vi "Begin.vi"(11 "Image Size":T1=enum."160x120") -> (0 "error out":errorcluster)   [LabVIEW 2012]
doc: "Called before other user functions, this VI is expected to open initial I/O refnums, load in file data, and do all program initialization. Notice that the <B>error out</B> terminal is simply used for data flow. Wiring it to other structures or subVIs ensures that this VI runs first."
uses:
  <vilib>/Rock Robotics/WPI/Camera/WPI_CameraImageSize.ctl
  <vilib>/Rock Robotics/WPI/Camera/WPI_CameraWhite Balance Values.ctl
  <vilib>/Rock Robotics/WPI/Camera/WPI_CameraExposure Values.ctl
  <vilib>/Rock Robotics/WPI/Camera/WPI_CameraFrameRate.ctl
  <vilib>/Rock Robotics/WPI/DriverStation/WPI_DriverStationRobotMode2.ctl
  <vilib>/Rock Robotics/WPI/Joystick/WPI_JoystickDeviceEnum.ctl
  <vilib>/Rock Robotics/WPI/CAN/Jaguar/SubVIs/WPI_CANJaguar_ControlMode.ctl
  <vilib>/Rock Robotics/WPI/CAN/Jaguar/SubVIs/WPI_CANJaguar_SpeedReference.ctl
  <vilib>/Rock Robotics/WPI/CAN/Jaguar/SubVIs/WPI_CANJaguar_PositionReference.ctl
  Robot Global Data.vi
  <vilib>/Rock Robotics/WPI/MotorControl/WPI_MotorControlOpenCANJaguar.vi
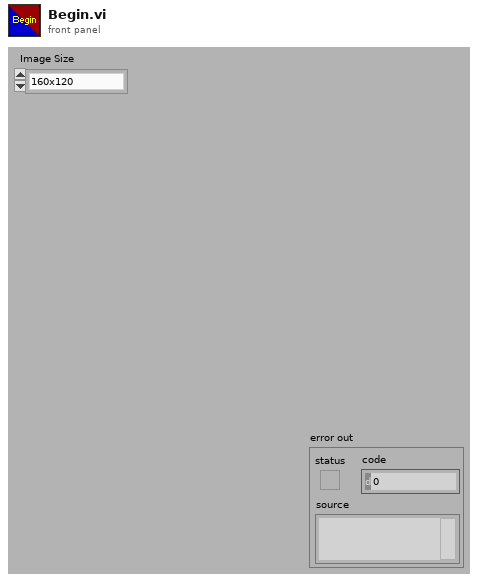
[diagram p1: front panel]
types:
  T1 = typedef "WPI_CameraImageSize.ctl" = enum16{"640x480", "320x240", "160x120"}
  T2 = typedef "WPI_JoystickDeviceEnum.ctl" = enum16{"USB 1", "USB 2", "USB 3", "USB 4", "Kinect 1", "Kinect 2"}
  T3 = typedef "WPI_CANJaguar_PositionReference.ctl" = u8
  T4 = typedef "WPI_CANJaguar_ControlMode.ctl" = enum8{"Percent VBus", "Current", "Speed", "Position", "Voltage"}
  T5 = typedef "WPI_CANJaguar_SpeedReference.ctl" = u8
  T6 = typedef "WPI_DriverStationRobotMode2.ctl" = enum16{"Autonomous Disabled", "Autonomous Enabled", "Teleop Disabled", "Teleop Enabled", "Timeout", "Finish", "Test Disabled", "Test Enabled"}
  T7 = typedef "WPI_CameraFrameRate.ctl" = u32
  T8 = typedef "WPI_CameraExposure Values.ctl" = enum16{"Auto", "Flicker-free 50 Hz", "Flicker-free 60 Hz", "Hold current"}
  T9 = typedef "WPI_CameraWhite Balance Values.ctl" = enum16{"Auto", "Fixed indoor", "Fixed outdoor 1", "Fixed outdoor 2", "Fixed fluorescent 1", "Fixed fluorescent 2", "Hold current"}
  T10 = typedef "WPI_MotorControlDeviceRef.ctl" = cluster{"DeviceStatus":errorcluster, "Type":enum16{"PWM", "CAN"}, "PWM":cluster{"Digital Module":T11, "PWM Channel":T12, "DeadBand":T13}, "CAN":cluster{"Device Number":u8, "Control Mode":T4, "Semaphore":T14, "Max Vout":dbl}, "Invert":bool, "TransformRef":T15, "InvTransformRef":T15}
  T11 = typedef "FPGA_TypedefDigitalModule.ctl" = enum16{"Digital Module 1", "Digital Module 2"}
  T12 = typedef "FPGA_DIOPWMChannel.ctl" = enum8{"PWM 1", "PWM 2", "PWM 3", "PWM 4", "PWM 5", "PWM 6", "PWM 7", "PWM 8", "PWM 9", "PWM 10", "Invalid"}
  T13 = typedef "WPI_PWMDeadband.ctl" = cluster{"Name":string, "maxPositivePwm":i32, "minPositivePwm":i32, "centerPwm":i32, "maxNegativePwm":i32, "minNegativePwm":i32, "angularRange":u16}
  T14 = typedef "Semaphore RefNum" = refnum<k1>
  T15 = typedef "WPI_PWMTransform_ConPane.ctl" = refnum<vi>
  T16 = typedef "WPI_JoystickDevRef.ctl" = cluster{"Device":T2}
  T17 = typedef "WPI_CameraDevRef.ctl" = cluster{"Camera Address":string, "CameraStatus":errorcluster, "Acquire Image Notifier":refnum<notifier>}
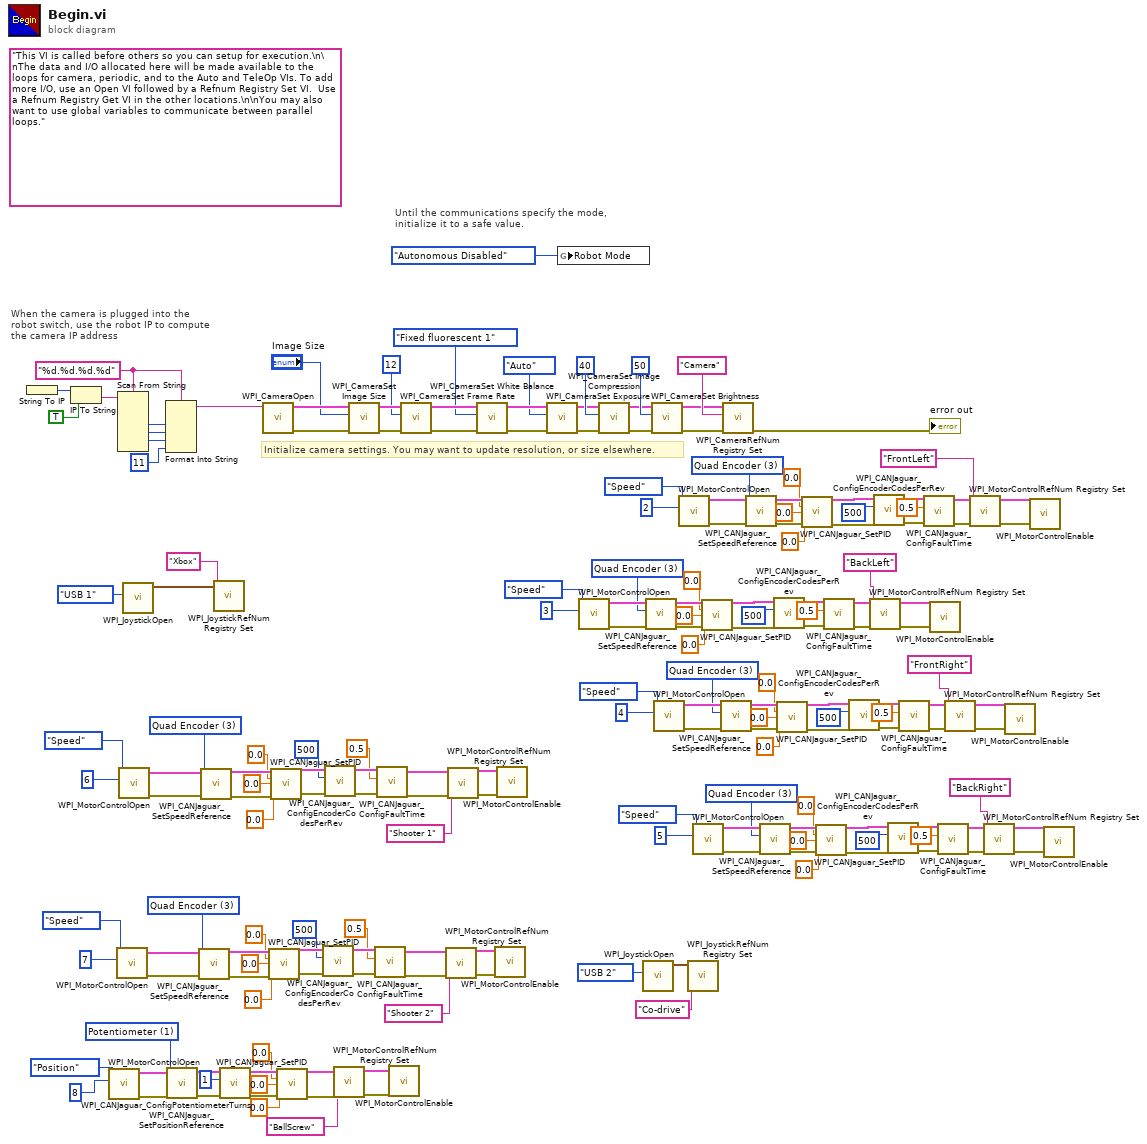
[diagram p0: block diagram]
diagram:
  w17 = T3 1 items=["Quad Encoder"=0, "Potentiometer"=1, "None"=255] ("Position Reference")
  w38 = T5 3 items=["Encoder"=0, "Inv Encoder"=2, "Quad Encoder"=3, "None"=255] ("Speed Reference")
  w59 = T5 3 items=["Encoder"=0, "Inv Encoder"=2, "Quad Encoder"=3, "None"=255] ("Speed Reference")
  w65 = T5 3 items=["Encoder"=0, "Inv Encoder"=2, "Quad Encoder"=3, "None"=255] ("Speed Reference")
  w86 = T5 3 items=["Encoder"=0, "Inv Encoder"=2, "Quad Encoder"=3, "None"=255] ("Speed Reference")
  w107 = T5 3 items=["Encoder"=0, "Inv Encoder"=2, "Quad Encoder"=3, "None"=255] ("Speed Reference")
  w143 = T5 3 items=["Encoder"=0, "Inv Encoder"=2, "Quad Encoder"=3, "None"=255] ("Speed Reference")
  w154 = "%d.%d.%d.%d" ("format string")
  (unwired) "This VI is called before others so you can setup for execution.\n\nThe data and I/O allocated here will be made available to the loops for camera, periodic, and to the Auto and TeleOp VIs. To add more I/O, use an Open VI followed by a Refnum Registry Set VI.  Use a Refnum Registry Get VI in the other locations.\n\nYou may also want to use global variables to communicate between parallel loops."
  # "Until the communications specify the mode,\ninitialize it to a safe value."
  # "When the camera is plugged into the\nrobot switch, use the robot IP to compute\nthe camera IP address"
  # "Initialize camera settings. You may want to update resolution, or size elsewhere."
  n1 = String To IP() -> (0:w161:u32)  [unwired: 1 in]
  n2 = IP To String(1:TRUE ("dot notation? (F)"), 2:w161) -> (0:w159:string)
  n3 = call-poly <vilib>:"WPI_MotorControlOpen.vi"("Device Number"=u8 8, "Control Mode"=WPI_CANJaguar_ControlMode."Position") -> ("error out"=w19:errorcluster, "MotorControlDeviceRef"=w18:T10)  [unwired: 8 in]
  n4 = call-poly <vilib>:"WPI_MotorControlOpen.vi"("Device Number"=u8 7, "Control Mode"=WPI_CANJaguar_ControlMode."Speed") -> ("error out"=w39:errorcluster, "MotorControlDeviceRef"=w40:T10)  [unwired: 8 in]
  n5 = Scan From String(format string=w154, input string=w159) -> (output 1=w158:i32, output 2=w157:i32, output 3=w156:i32)  [unwired: 7 in, 3 out]
  n6 = call-poly <vilib>:"WPI_MotorControlOpen.vi"("Device Number"=u8 6, "Control Mode"=WPI_CANJaguar_ControlMode."Speed") -> ("error out"=w60:errorcluster, "MotorControlDeviceRef"=w61:T10)  [unwired: 8 in]
  n7 = call <vilib>:"WPI_JoystickOpen.vi"("JoystickDevice"=WPI_JoystickDeviceEnum."USB 1") -> ("JoystickDevRef"=w150:T16)  [unwired: 10 in]
  n8 = Format Into String(format string=w154, w158, w157, w156, 11 ("Compression")) -> (resulting string=w152:string)  [unwired: 2 in, 1 out]
  n9 = call <vilib>:"WPI_CANJaguar_SetPositionReference.vi"("error in (no error)"=w19, "Position Reference"=w17, "CAN Jaguar Ref"=w18) -> ("error out"=w16:errorcluster, "CAN Jaguar Ref Out"=w15:T10)  [unwired: 7 in]
  n10 = call <vilib>:"WPI_CANJaguar_SetSpeedReference.vi"("error in (no error)"=w39, "Speed Reference"=w38, "CAN Jaguar Ref"=w40) -> ("error out"=w36:errorcluster, "CAN Jaguar Ref Out"=w37:T10)  [unwired: 7 in]
  n11 = call <vilib>:"WPI_CANJaguar_SetSpeedReference.vi"("error in (no error)"=w60, "Speed Reference"=w59, "CAN Jaguar Ref"=w61) -> ("error out"=w57:errorcluster, "CAN Jaguar Ref Out"=w58:T10)  [unwired: 7 in]
  n12 = call <vilib>:"WPI_JoystickRefNum Registry Set.vi"("refnum name"="Xbox", "JoystickDevRef"=w150) -> ()  [unwired: 8 in, 2 out]
  n13 = call <vilib>:"WPI_CANJaguar_ConfigPotentiometerTurns.vi"("error in (no error)"=w16, "Potentiometer Turns"=u16 1, "CAN Jaguar Ref"=w15) -> ("error out"=w12:errorcluster, "CAN Jaguar Ref Out"=w13:T10)  [unwired: 7 in]
  n14 = call <vilib>:"WPI_CameraOpen.vi"("Camera Address"=w152) -> ("error out"=w173:errorcluster, "CameraDevRef"=w174:T17)  [unwired: 1 in, 8 out]
  n15 = call <vilib>:"WPI_CANJaguar_SetPID.vi"("CAN Jaguar Ref"=w37, "P"=0.0, "I"=0.0, "D"=0.0, "error in (no error)"=w36) -> ("CAN Jaguar Ref Out"=w32:T10, "error out"=w31:errorcluster)  [unwired: 9 in]
  n16 = call <vilib>:"WPI_CANJaguar_SetPID.vi"("CAN Jaguar Ref"=w58, "P"=0.0, "I"=0.0, "D"=0.0, "error in (no error)"=w57) -> ("CAN Jaguar Ref Out"=w53:T10, "error out"=w52:errorcluster)  [unwired: 9 in]
  n17 = call <vilib>:"WPI_CANJaguar_SetPID.vi"("CAN Jaguar Ref"=w13, "P"=0.0, "I"=0.0, "D"=0.0, "error in (no error)"=w12) -> ("CAN Jaguar Ref Out"=w7:T10, "error out"=w8:errorcluster)  [unwired: 9 in]
  n18 = call <vilib>:"WPI_CANJaguar_ConfigEncoderCodesPerRev.vi"("error in (no error)"=w31, "Encoder Codes Per Rev"=u16 500, "CAN Jaguar Ref"=w32) -> ("error out"=w29:errorcluster, "CAN Jaguar Ref Out"=w28:T10)  [unwired: 7 in]
  n19 = call <vilib>:"WPI_CANJaguar_ConfigEncoderCodesPerRev.vi"("error in (no error)"=w52, "Encoder Codes Per Rev"=u16 500, "CAN Jaguar Ref"=w53) -> ("error out"=w50:errorcluster, "CAN Jaguar Ref Out"=w49:T10)  [unwired: 7 in]
  n20 = call <vilib>:"WPI_MotorControlRefNum Registry Set.vi"("error in (no error)"=w8, "refnum name"="BallScrew", "MotorControlDevRef"=w7) -> ("error out"=w6:errorcluster, "MotorControlDevRef"=w5:T10)  [unwired: 7 in]
  n21 = call <vilib>:"WPI_CameraSet Image Size.vi"("error in (no error)"=w173, "Image Size"="Image Size", "CameraDevRef"=w174) -> ("error out"=w172:errorcluster, "CameraDevRef Out"=w175:T17)  [unwired: 7 out]
  n22 = call <vilib>:"WPI_CANJaguar_ConfigFaultTime.vi"("error in (no error)"=w29, "Fault Time (s)"=0.5, "CAN Jaguar Ref"=w28) -> ("error out"=w24:errorcluster, "CAN Jaguar Ref Out"=w25:T10)  [unwired: 7 in]
  n23 = call <vilib>:"WPI_CANJaguar_ConfigFaultTime.vi"("error in (no error)"=w50, "Fault Time (s)"=0.5, "CAN Jaguar Ref"=w49) -> ("error out"=w45:errorcluster, "CAN Jaguar Ref Out"=w46:T10)  [unwired: 7 in]
  n24 = call <vilib>:"WPI_MotorControlEnable.vi"("error in (no error)"=w6, "CAN Jaguar Ref"=w5) -> ()  [unwired: 8 in, 2 out]
  n25 = call <vilib>:"WPI_CameraSet Frame Rate.vi"("error in (no error)"=w172, "Frame Rate (fps)"=T7 12, "CameraDevRef"=w175) -> ("error out"=w171:errorcluster, "CameraDevRef Out"=w177:T17)  [unwired: 7 out]
  n26 = call <vilib>:"WPI_MotorControlRefNum Registry Set.vi"("error in (no error)"=w24, "refnum name"="Shooter 2", "MotorControlDevRef"=w25) -> ("error out"=w22:errorcluster, "MotorControlDevRef"=w23:T10)  [unwired: 7 in]
  n27 = call <vilib>:"WPI_MotorControlRefNum Registry Set.vi"("error in (no error)"=w45, "refnum name"="Shooter 1", "MotorControlDevRef"=w46) -> ("error out"=w43:errorcluster, "MotorControlDevRef"=w44:T10)  [unwired: 7 in]
  n28 = call <vilib>:"WPI_CameraSet White Balance.vi"("error in (no error)"=w171, "White Balance"=WPI_CameraWhite_Balance_Values."Fixed fluorescent 1", "CameraDevRef"=w177) -> ("error out"=w170:errorcluster, "CameraDevRef Out"=w176:T17)  [unwired: 7 out]
  n29 = call <vilib>:"WPI_MotorControlEnable.vi"("error in (no error)"=w22, "CAN Jaguar Ref"=w23) -> ()  [unwired: 8 in, 2 out]
  n30 = call <vilib>:"WPI_MotorControlEnable.vi"("error in (no error)"=w43, "CAN Jaguar Ref"=w44) -> ()  [unwired: 8 in, 2 out]
  n31 = call <vilib>:"WPI_CameraSet Exposure.vi"("error in (no error)"=w170, "Exposure"=WPI_CameraExposure_Values."Auto", "CameraDevRef"=w176) -> ("error out"=w169:errorcluster, "CameraDevRef Out"=w179:T17)  [unwired: 7 out]
  n32 = global write "Robot Global Data.vi" "Robot Mode"(WPI_DriverStationRobotMode2."Autonomous Disabled" ("Robot Mode")) -> ()
  n33 = call-poly <vilib>:"WPI_MotorControlOpen.vi"("Device Number"=u8 3, "Control Mode"=WPI_CANJaguar_ControlMode."Speed") -> ("error out"=w123:errorcluster, "MotorControlDeviceRef"=w124:T10)  [unwired: 8 in]
  n34 = call <vilib>:"WPI_CameraSet Image Compression.vi"("error in (no error)"=w169, "Compression"=40, "CameraDevRef"=w179) -> ("error out"=w168:errorcluster, "CameraDevRef Out"=w178:T17)  [unwired: 7 out]
  n35 = call <vilib>:"WPI_JoystickOpen.vi"("JoystickDevice"=WPI_JoystickDeviceEnum."USB 2") -> ("JoystickDevRef"=w2:T16)  [unwired: 10 in]
  n36 = call <vilib>:"WPI_CANJaguar_SetSpeedReference.vi"("error in (no error)"=w123, "Speed Reference"=w107, "CAN Jaguar Ref"=w124) -> ("error out"=w121:errorcluster, "CAN Jaguar Ref Out"=w122:T10)  [unwired: 7 in]
  n37 = call <vilib>:"WPI_CameraSet Brightness.vi"("error in (no error)"=w168, "Brightness"=50, "CameraDevRef"=w178) -> ("error out"=w166:errorcluster, "CameraDevRef Out"=w167:T17)  [unwired: 7 out]
  n38 = call-poly <vilib>:"WPI_MotorControlOpen.vi"("Device Number"=u8 4, "Control Mode"=WPI_CANJaguar_ControlMode."Speed") -> ("error out"=w102:errorcluster, "MotorControlDeviceRef"=w103:T10)  [unwired: 8 in]
  n39 = call-poly <vilib>:"WPI_MotorControlOpen.vi"("Device Number"=u8 2, "Control Mode"=WPI_CANJaguar_ControlMode."Speed") -> ("error out"=w144:errorcluster, "MotorControlDeviceRef"=w145:T10)  [unwired: 8 in]
  n40 = call <vilib>:"WPI_JoystickRefNum Registry Set.vi"("refnum name"="Co-drive", "JoystickDevRef"=w2) -> ()  [unwired: 8 in, 2 out]
  n41 = call-poly <vilib>:"WPI_MotorControlOpen.vi"("Device Number"=u8 5, "Control Mode"=WPI_CANJaguar_ControlMode."Speed") -> ("error out"=w81:errorcluster, "MotorControlDeviceRef"=w82:T10)  [unwired: 8 in]
  n42 = call <vilib>:"WPI_CANJaguar_SetPID.vi"("CAN Jaguar Ref"=w122, "P"=0.0, "I"=0.0, "D"=0.0, "error in (no error)"=w121) -> ("CAN Jaguar Ref Out"=w116:T10, "error out"=w117:errorcluster)  [unwired: 9 in]
  n43 = call <vilib>:"WPI_CANJaguar_SetSpeedReference.vi"("error in (no error)"=w102, "Speed Reference"=w86, "CAN Jaguar Ref"=w103) -> ("error out"=w100:errorcluster, "CAN Jaguar Ref Out"=w101:T10)  [unwired: 7 in]
  n44 = call <vilib>:"WPI_CameraRefNum Registry Set.vi"("error in (no error)"=w166, "refnum name"="Camera", "CameraDevRef"=w167) -> ("error out"=→"error out":errorcluster)  [unwired: 8 out]
  n45 = call <vilib>:"WPI_CANJaguar_SetSpeedReference.vi"("error in (no error)"=w144, "Speed Reference"=w143, "CAN Jaguar Ref"=w145) -> ("error out"=w141:errorcluster, "CAN Jaguar Ref Out"=w142:T10)  [unwired: 7 in]
  n46 = call <vilib>:"WPI_CANJaguar_SetSpeedReference.vi"("error in (no error)"=w81, "Speed Reference"=w65, "CAN Jaguar Ref"=w82) -> ("error out"=w79:errorcluster, "CAN Jaguar Ref Out"=w80:T10)  [unwired: 7 in]
  n47 = call <vilib>:"WPI_CANJaguar_ConfigEncoderCodesPerRev.vi"("error in (no error)"=w117, "Encoder Codes Per Rev"=u16 500, "CAN Jaguar Ref"=w116) -> ("error out"=w111:errorcluster, "CAN Jaguar Ref Out"=w112:T10)  [unwired: 7 in]
  n48 = call <vilib>:"WPI_CANJaguar_SetPID.vi"("CAN Jaguar Ref"=w101, "P"=0.0, "I"=0.0, "D"=0.0, "error in (no error)"=w100) -> ("CAN Jaguar Ref Out"=w95:T10, "error out"=w96:errorcluster)  [unwired: 9 in]
  n49 = call <vilib>:"WPI_CANJaguar_SetPID.vi"("CAN Jaguar Ref"=w142, "P"=0.0, "I"=0.0, "D"=0.0, "error in (no error)"=w141) -> ("CAN Jaguar Ref Out"=w136:T10, "error out"=w137:errorcluster)  [unwired: 9 in]
  n50 = call <vilib>:"WPI_CANJaguar_SetPID.vi"("CAN Jaguar Ref"=w80, "P"=0.0, "I"=0.0, "D"=0.0, "error in (no error)"=w79) -> ("CAN Jaguar Ref Out"=w74:T10, "error out"=w75:errorcluster)  [unwired: 9 in]
  n51 = call <vilib>:"WPI_CANJaguar_ConfigFaultTime.vi"("error in (no error)"=w111, "Fault Time (s)"=0.5, "CAN Jaguar Ref"=w112) -> ("error out"=w109:errorcluster, "CAN Jaguar Ref Out"=w110:T10)  [unwired: 7 in]
  n52 = call <vilib>:"WPI_CANJaguar_ConfigEncoderCodesPerRev.vi"("error in (no error)"=w96, "Encoder Codes Per Rev"=u16 500, "CAN Jaguar Ref"=w95) -> ("error out"=w90:errorcluster, "CAN Jaguar Ref Out"=w91:T10)  [unwired: 7 in]
  n53 = call <vilib>:"WPI_MotorControlRefNum Registry Set.vi"("error in (no error)"=w109, "refnum name"="BackLeft", "MotorControlDevRef"=w110) -> ("error out"=w114:errorcluster, "MotorControlDevRef"=w113:T10)  [unwired: 7 in]
  n54 = call <vilib>:"WPI_CANJaguar_ConfigEncoderCodesPerRev.vi"("error in (no error)"=w137, "Encoder Codes Per Rev"=u16 500, "CAN Jaguar Ref"=w136) -> ("error out"=w130:errorcluster, "CAN Jaguar Ref Out"=w131:T10)  [unwired: 7 in]
  n55 = call <vilib>:"WPI_CANJaguar_ConfigEncoderCodesPerRev.vi"("error in (no error)"=w75, "Encoder Codes Per Rev"=u16 500, "CAN Jaguar Ref"=w74) -> ("error out"=w69:errorcluster, "CAN Jaguar Ref Out"=w70:T10)  [unwired: 7 in]
  n56 = call <vilib>:"WPI_CANJaguar_ConfigFaultTime.vi"("error in (no error)"=w90, "Fault Time (s)"=0.5, "CAN Jaguar Ref"=w91) -> ("error out"=w88:errorcluster, "CAN Jaguar Ref Out"=w89:T10)  [unwired: 7 in]
  n57 = call <vilib>:"WPI_CANJaguar_ConfigFaultTime.vi"("error in (no error)"=w130, "Fault Time (s)"=0.5, "CAN Jaguar Ref"=w131) -> ("error out"=w128:errorcluster, "CAN Jaguar Ref Out"=w129:T10)  [unwired: 7 in]
  n58 = call <vilib>:"WPI_MotorControlEnable.vi"("error in (no error)"=w114, "CAN Jaguar Ref"=w113) -> ()  [unwired: 8 in, 2 out]
  n59 = call <vilib>:"WPI_CANJaguar_ConfigFaultTime.vi"("error in (no error)"=w69, "Fault Time (s)"=0.5, "CAN Jaguar Ref"=w70) -> ("error out"=w67:errorcluster, "CAN Jaguar Ref Out"=w68:T10)  [unwired: 7 in]
  n60 = call <vilib>:"WPI_MotorControlRefNum Registry Set.vi"("error in (no error)"=w88, "refnum name"="FrontRight", "MotorControlDevRef"=w89) -> ("error out"=w93:errorcluster, "MotorControlDevRef"=w92:T10)  [unwired: 7 in]
  n61 = call <vilib>:"WPI_MotorControlRefNum Registry Set.vi"("error in (no error)"=w128, "refnum name"="FrontLeft", "MotorControlDevRef"=w129) -> ("error out"=w133:errorcluster, "MotorControlDevRef"=w132:T10)  [unwired: 7 in]
  n62 = call <vilib>:"WPI_MotorControlRefNum Registry Set.vi"("error in (no error)"=w67, "refnum name"="BackRight", "MotorControlDevRef"=w68) -> ("error out"=w72:errorcluster, "MotorControlDevRef"=w71:T10)  [unwired: 7 in]
  n63 = call <vilib>:"WPI_MotorControlEnable.vi"("error in (no error)"=w93, "CAN Jaguar Ref"=w92) -> ()  [unwired: 8 in, 2 out]
  n64 = call <vilib>:"WPI_MotorControlEnable.vi"("error in (no error)"=w133, "CAN Jaguar Ref"=w132) -> ()  [unwired: 8 in, 2 out]
  n65 = call <vilib>:"WPI_MotorControlEnable.vi"("error in (no error)"=w72, "CAN Jaguar Ref"=w71) -> ()  [unwired: 8 in, 2 out]
